vi "Finalize Settings.vi"(8 "error in (no error)":errorcluster, 10 "settings version":T3, 11 "configuration":T1={"name"="Channel", "units"="V", "engine data type"=enum."DBL", "string data type"=enum."DBL", "string offset"=0} {"string offset" format="%d bytes"}) -> (0 "error out":errorcluster, 2 "settings version":T3, 3 "settings":cluster{"key":string, "value":string}[](array[cluster]))   [LabVIEW 2019, in "DSF Core.lvlib" / "Channel Configuration.lvclass"]
uses:
  Channel Configuration.lvclass
  Typedefs/DSF Version Info.ctl
  Typedefs/Core Channel Configuration.ctl
  Typedefs/DSF Data Type.ctl
  DSF Core.lvlib
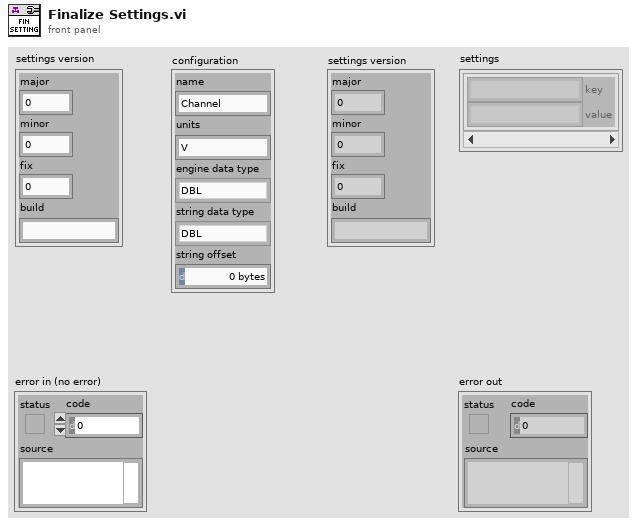
[diagram p1: front panel]
types:
  T1 = typedef "DSF Core.lvlib/Channel Configuration.lvclass/Core Channel Configuration.ctl" = cluster{"name":string, "units":string, "engine data type":T2, "string data type":T2, "string offset":u64}
  T2 = typedef "DSF Core.lvlib/DSF Data Type.ctl" = enum8{"Bool", "SGL", "DBL", "I8", "I16", "I32", "I64", "U8", "U16", "U32", "U64"}
  T3 = typedef "DSF Core.lvlib/DSF Version Info.ctl" = cluster{"major":u32, "minor":u32, "fix":u32, "build":string}
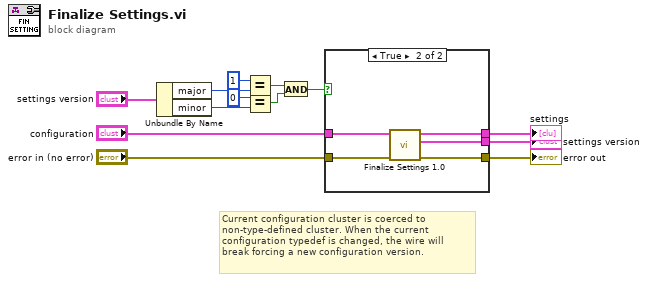
[diagram p0: block diagram]
diagram:
  # "Current configuration cluster is coerced to non-type-defined cluster. When the current configuration typedef is changed, the wire will break forcing a new configuration version."
  n1 = Unbundle By Name("settings version") -> ("major"=w9:u32, "minor"=w6:u32)
  n2 = Equal?(x=u32 1, y=w9) -> (x = y?=w4:bool)
  n3 = Equal?(x=u32 0, y=w6) -> (x = y?=w3:bool)
  n4 = And(x=w4, y=w3) -> (x .and. y?=w5:bool)
  n5 = case shown="True" w5 {
    tunnel: [w14 w19] -> w13
    tunnel: "error in (no error)" -> [w14 w18]
    tunnel: "configuration" -> [_ w15]
    tunnel: [_ w17] -> w11
    tunnel: [_ w16] -> w2
    frame False {
      # "#TODO\nUnknown version. Error."
    }
    frame True {
      n6 = call "Finalize Settings 1.0.vi"("error in (no error)"=w18, "configuration 1.0"=w15) -> ("error out"=w19:errorcluster, "settings version"=w16:T3, "settings 1.0"=w17:cluster{"key":string, "value":string}[])  [unwired: 7 in]
    }
  }
  "error out" <- w13
  "settings" <- w11
  "settings version" <- w2
